vi "Retest check.vi"(0 "SerialNumber":string, 1 "Variant":string) -> (12 "Number of passes":u8, 13 "Number of Fails":u8, 14 "index of element":i32, 15 "Already tested":bool, 16 "SerialNumber only of digits":bool, 17 "Already passed":bool, 18 "Max Fail":bool)   [LabVIEW 2023]
uses:
  <vilib>/Utility/file.llb/Read Delimited Spreadsheet (I64).vi
panel:
  out "output array":i64[](array[numeric])
  out "subarray 2":i64[][](array[numeric])
  out "subarray":i64[][](array[numeric])
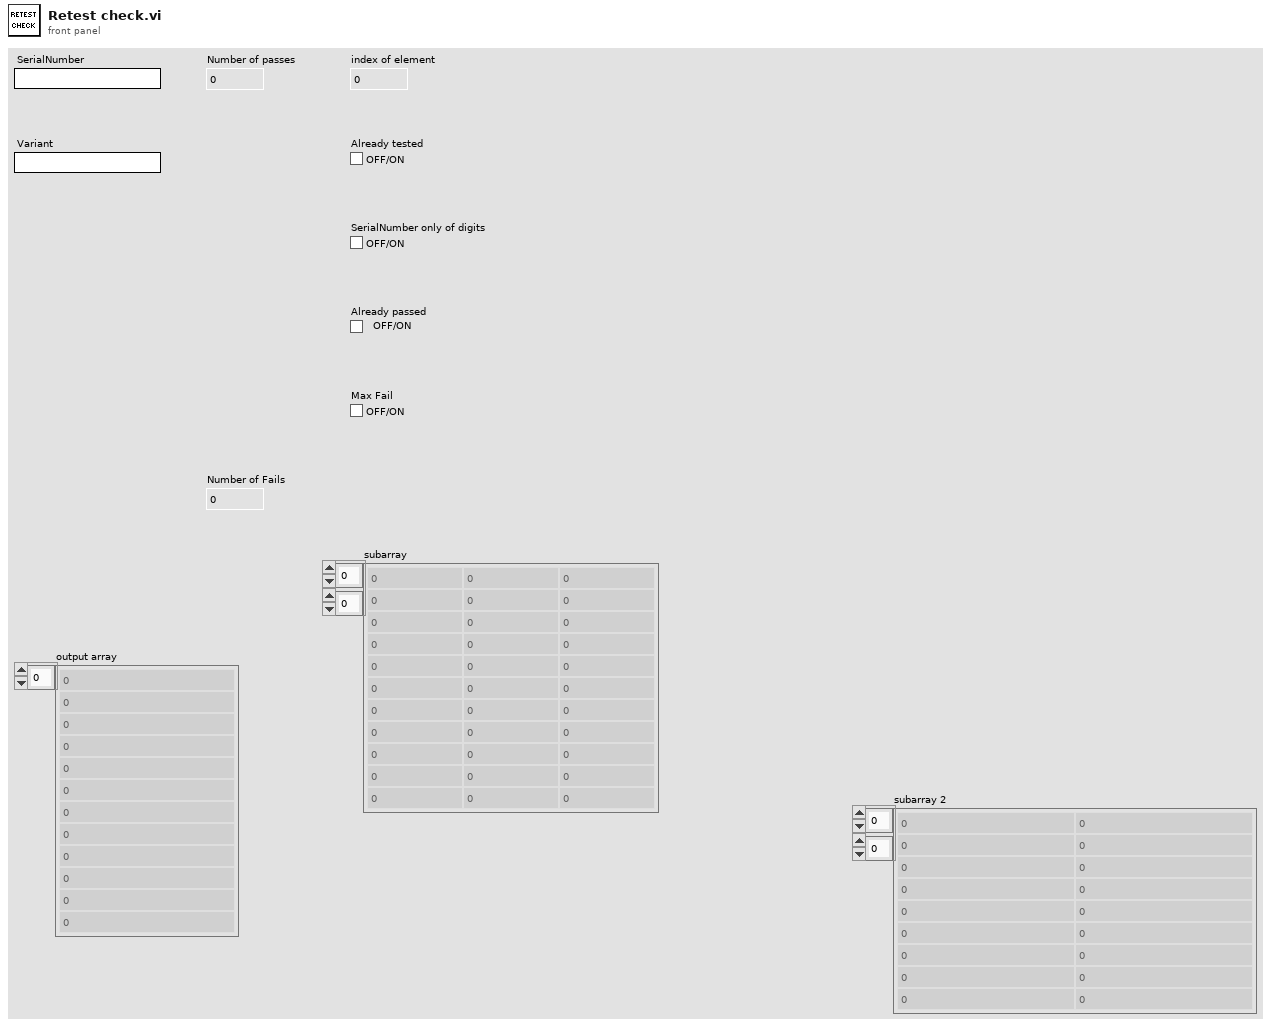
[diagram p1: front panel]
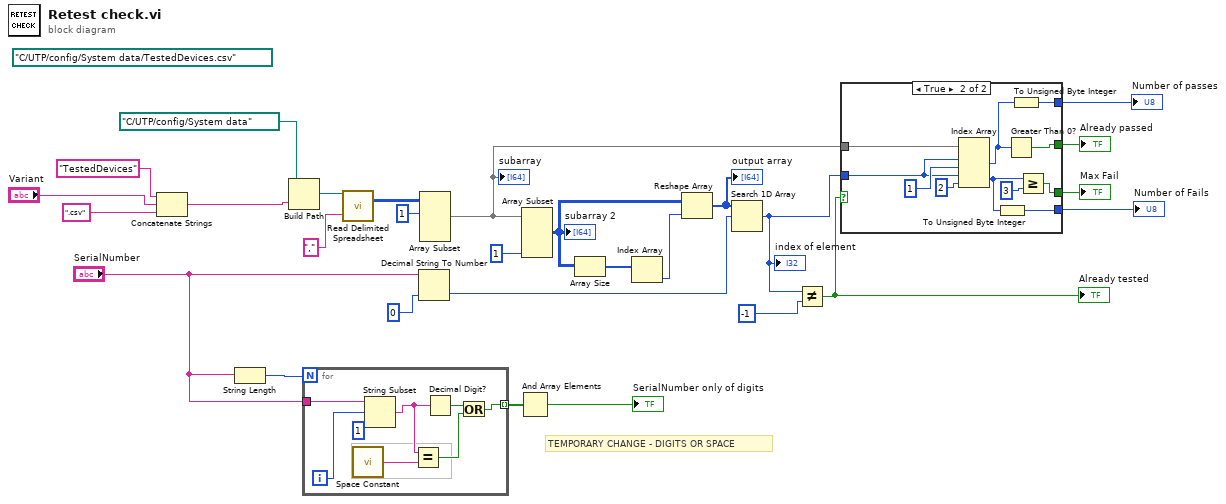
[diagram p0: block diagram]
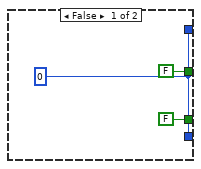
[diagram p2: hidden frame]
diagram:
  (unwired) path "C:/UTP/config/System data/TestedDevices.csv" ("file path (dialog if empty)")
  # "TEMPORARY CHANGE - DIGITS OR SPACE"
  n1 = Concatenate Strings("TestedDevices" ("string"), "Variant", ".csv" ("string")) -> (w3:string)
  n2 = String Length(string="SerialNumber") -> (length=w11:i32)
  n3 = Build Path(base path=path "C:/UTP/config/System data" ("file path (dialog if empty)"), name or relative path=w3) -> (appended path=w2:path)
  n4 = for {
    N: w11 -> [_]
    tunnel: [w29] -> w13 mode=indexing
    tunnel: "SerialNumber" -> [w36]
    i -> [w35]
    n5 = call <vilib>:"Space Constant.vi"() -> ("String"=w32:string)
    n6 = String Subset(string=w36, offset (0)=w35, length (rest)=1 ("length (rest)")) -> (substring=w33:string)
    n7 = Equal?(x=w33, y=w32) -> (x = y?=w30:bool)
    n8 = Decimal Digit?(1:w33) -> (0:w31:bool)
    n9 = Or(x=w31, y=w30) -> (x .or. y?=w29:bool)
  }
  n10 = call-poly <vilib>:"Read Delimited Spreadsheet.vi"("file path (dialog if empty)"=w2, "delimiter (\\t)"="," ("delimiter (\\t)")) -> ("all rows"=w17:i64[][])  [unwired: 8 in, 5 out]
  n11 = Decimal String To Number(string="SerialNumber", default (0L)=i64 0 ("default (0 I32)")) -> (number=w14:i64)  [unwired: 1 in, 1 out]
  n12 = Array Subset(array=w17, index (row)=1 ("index")) -> (w16:i64[][])  [unwired: 3 in]
  "subarray" <- w16
  n13 = And Array Elements(Boolean array=w13) -> (logical AND=→"SerialNumber only of digits":bool)
  n14 = Array Subset(array=w16, length (col)=1 ("length")) -> (w25:i64[][])  [unwired: 3 in]
  "subarray 2" <- w25
  n15 = Array Size(array=w25) -> (size(s)=w24:i32[])
  n16 = Index Array(array=w24) -> (element=w23:i32)  [unwired: 1 in]
  n17 = Reshape Array(w25, w23) -> (w21:i64[])
  "output array" <- w21
  n18 = Search 1D Array(1D array=w21, element=w14) -> (index of element=w20:i32)  [unwired: 1 in]
  "index of element" <- w20
  n19 = Not Equal?(x=w20, y=-1) -> (x != y?=w28:bool)
  "Already tested" <- w28
  n20 = case shown="True" w28 {
    tunnel: w16 -> [_ w50]
    tunnel: w20 -> [_ w47]
    tunnel: [FALSE w45] -> w19
    tunnel: [FALSE w44] -> w18
    tunnel: [w37 w42] -> w9
    tunnel: [w37 w40] -> w8
    frame False {
      w37 = u8 0 ("Numeric")
    }
    frame True {
      n21 = Index Array(array=w50, index (row) #1=w47, index (col) #1=1 ("index (col)"), index (row) #2=w47, index (col) #2=2 ("index (col)")) -> (element #1=w43:i64, element #2=w41:i64)
      n22 = To Unsigned Byte Integer(number=w41) -> (unsigned 8bit integer=w40:u8)
      n23 = Greater Than 0?(x=w43) -> (x > 0?=w45:bool)
      n24 = To Unsigned Byte Integer(number=w43) -> (unsigned 8bit integer=w42:u8)
      n25 = Greater Or Equal?(x=w41, y=i64 3) -> (x >= y?=w44:bool)
    }
  }
  "Already passed" <- w19
  "Max Fail" <- w18
  "Number of passes" <- w9
  "Number of Fails" <- w8
